vi "双路双通通断器（VAR）.vi"(7 "默认值":variant, 9 "直通？":bool=TRUE, 10 "Y_In":variant, 11 "X_In":variant) -> (2 "Y_Out":variant, 3 "X_Out":variant)   [LabVIEW 2011]
doc: "功能：\n\n返回一个枚举，表明输入数的范围，用于三段比较。\n\n\nCSXCS_366创建。"
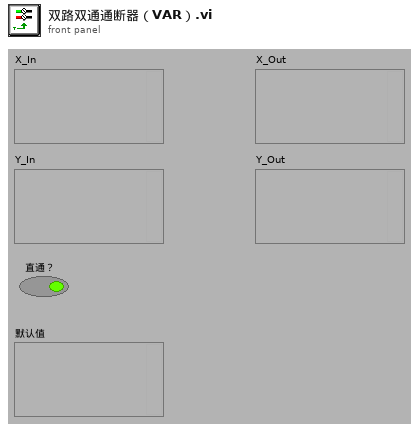
[diagram p1: front panel]
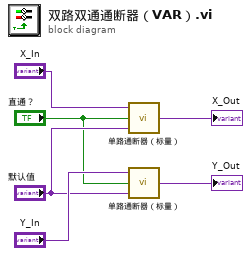
[diagram p0: block diagram]
diagram:
  n1 = call-poly "单路通断器（标量）.vi"("默认值"="默认值", "直通？"="直通？", "X_In"="X_In") -> ("X_Out"=→"X_Out":variant)
  n2 = call-poly "单路通断器（标量）.vi"("默认值"="默认值", "直通？"="直通？", "X_In"="Y_In") -> ("X_Out"=→"Y_Out":variant)
